vi "Post-Install Custom Action.vi"(10 "Variant":variant) -> (0 "error out":errorcluster)   [LabVIEW 2013]
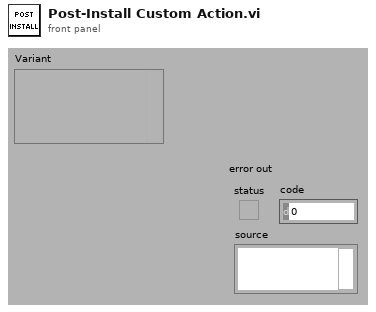
[diagram p1: front panel]
types:
  T1 = enum32{"invalid lock state", "Not Locked", "Locked (No Password)", "Password-protected"}
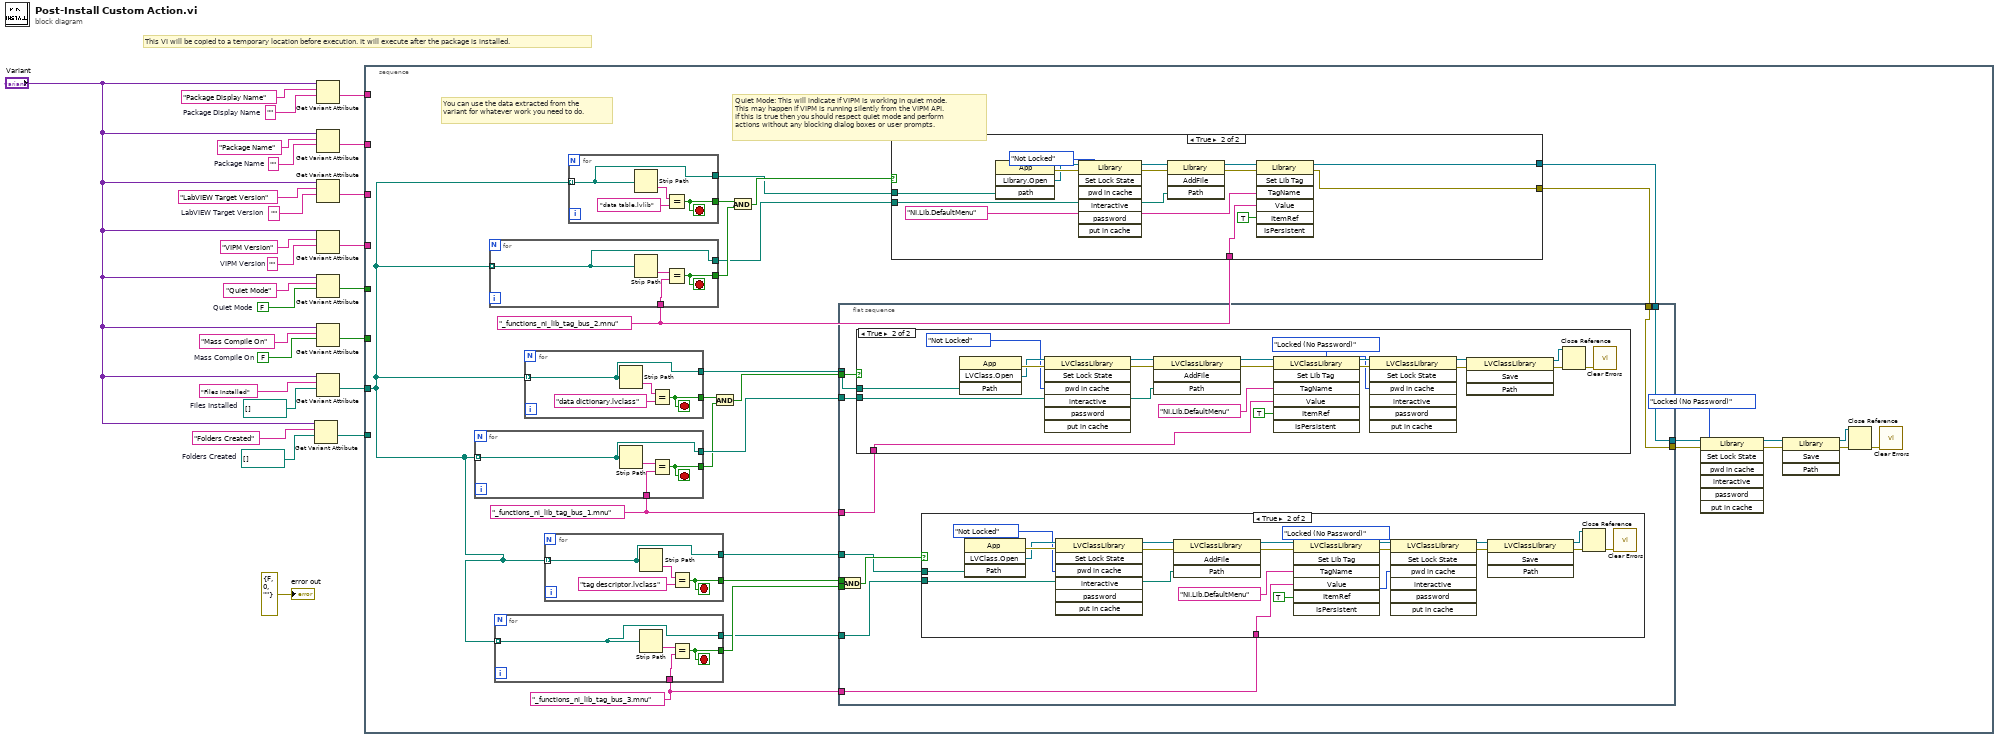
[diagram p0: block diagram]
diagram:
  w1 = path[] []  # Folders Created
  w2 = path[] []  # Files Installed
  w8 = FALSE  # Mass Compile On
  w9 = ""  # Package Display Name
  w16 = FALSE  # Quiet Mode
  w19 = ""  # VIPM Version
  w21 = ""  # LabVIEW Target Version
  w23 = ""  # Package Name
  # "This VI will be copied to a temporary location before execution. It will execute after the package is installed."
  n1 = Get Variant Attribute(Variant="Variant", name="Folders Created", default value (empty Variant)=w1) -> (value=w6:path[])  [unwired: 1 in, 3 out]
  n2 = Get Variant Attribute(Variant="Variant", name="Package Display Name", default value (empty Variant)=w9) -> (value=w15:string)  [unwired: 1 in, 3 out]
  n3 = Get Variant Attribute(Variant="Variant", name="Package Name", default value (empty Variant)=w23) -> (value=w14:string)  [unwired: 1 in, 3 out]
  n4 = Get Variant Attribute(Variant="Variant", name="LabVIEW Target Version", default value (empty Variant)=w21) -> (value=w13:string)  [unwired: 1 in, 3 out]
  n5 = Get Variant Attribute(Variant="Variant", name="VIPM Version", default value (empty Variant)=w19) -> (value=w12:string)  [unwired: 1 in, 3 out]
  n6 = Get Variant Attribute(Variant="Variant", name="Quiet Mode", default value (empty Variant)=w16) -> (value=w11:bool)  [unwired: 1 in, 3 out]
  n7 = Get Variant Attribute(Variant="Variant", name="Mass Compile On", default value (empty Variant)=w8) -> (value=w10:bool)  [unwired: 1 in, 3 out]
  n8 = Get Variant Attribute(Variant="Variant", name="Files Installed", default value (empty Variant)=w2) -> (value=w5:path[])  [unwired: 1 in, 3 out]
  n9 = stacked-sequence {
    tunnel: w15 -> [_]
    tunnel: w14 -> [_]
    tunnel: w13 -> [_]
    tunnel: w12 -> [_]
    tunnel: w11 -> [_]
    tunnel: w10 -> [_]
    tunnel: w5 -> [w40]
    tunnel: w6 -> [_]
    frame #0 {
      w37 = "_functions_ni_lib_tag_bus_3.mnu" ("pattern")
      w38 = "_functions_ni_lib_tag_bus_1.mnu" ("pattern")
      w39 = "_functions_ni_lib_tag_bus_2.mnu" ("pattern")
      # "Quiet Mode: This will indicate if VIPM is working in quiet mode.\nThis may happen if VIPM is running silently from the VIPM API.\nIf this is true then you should respect quiet mode and perform\nactions without any blocking dialog boxes or user prompts."
      # "You can use the data extracted from the variant for whatever work you need to do."
      n10 = for {
        tunnel: w40 -> [w115] mode=indexing
        tunnel: [w115] -> w49
        tunnel: [w117] -> w45
        tunnel: w38 -> [w116]
        stop <- w117 stop-if-true
        n11 = Strip Path(path=w115) -> (name=w118:string)  [unwired: 1 out]
        n12 = Equal?(x=w118, y=w116) -> (x = y?=w117:bool)
      }
      n13 = for {
        tunnel: w40 -> [w137] mode=indexing
        tunnel: [w137] -> w50
        tunnel: [w139] -> w54
        tunnel: w39 -> [w138]
        stop <- w139 stop-if-true
        n14 = Strip Path(path=w137) -> (name=w140:string)  [unwired: 1 out]
        n15 = Equal?(x=w140, y=w138) -> (x = y?=w139:bool)
      }
      n16 = for {
        tunnel: w40 -> [w107] mode=indexing
        tunnel: [w107] -> w41
        tunnel: [w109] -> w44
        tunnel: w37 -> [w108]
        stop <- w109 stop-if-true
        n17 = Strip Path(path=w107) -> (name=w110:string)  [unwired: 1 out]
        n18 = Equal?(x=w110, y=w108) -> (x = y?=w109:bool)
      }
      n19 = for {
        tunnel: w40 -> [w119] mode=indexing
        tunnel: [w119] -> w48
        tunnel: [w120] -> w46
        stop <- w120 stop-if-true
        n20 = Strip Path(path=w119) -> (name=w121:string)  [unwired: 1 out]
        n21 = Equal?(x=w121, y="data dictionary.lvclass" ("pattern")) -> (x = y?=w120:bool)
      }
      n22 = for {
        tunnel: w40 -> [w111] mode=indexing
        tunnel: [w111] -> w42
        tunnel: [w112] -> w43
        stop <- w112 stop-if-true
        n23 = Strip Path(path=w111) -> (name=w113:string)  [unwired: 1 out]
        n24 = Equal?(x=w113, y="tag descriptor.lvclass" ("pattern")) -> (x = y?=w112:bool)
      }
      n25 = for {
        tunnel: w40 -> [w141] mode=indexing
        tunnel: [w141] -> w51
        tunnel: [w142] -> w53
        stop <- w142 stop-if-true
        n26 = Strip Path(path=w141) -> (name=w143:string)  [unwired: 1 out]
        n27 = Equal?(x=w143, y="data table.lvlib" ("pattern")) -> (x = y?=w142:bool)
      }
      n28 = And(x=w46, y=w45) -> (x .and. y?=w47:bool)
      n29 = And(x=w53, y=w54) -> (x .and. y?=w52:bool)
      n30 = flat-sequence {
        tunnel: w49 -> [w66]
        tunnel: w48 -> [w65]
        tunnel: w47 -> [w64]
        tunnel: w44 -> [w63]
        tunnel: w43 -> [w62]
        tunnel: w42 -> [w60]
        tunnel: w41 -> [w59]
        tunnel: w38 -> [w58]
        tunnel: w37 -> [w57]
        tunnel: w31 -> [w55]
        tunnel: [w56] -> w30
        tunnel: w29 -> [w56]
        tunnel: [w55] -> w28
        frame #0 {
          n31 = And(x=w62, y=w63) -> (x .and. y?=w61:bool)
          n32 = case shown="True" w64 {
            tunnel: w65 -> [_ w97]
            tunnel: w66 -> [_ w96]
            tunnel: w58 -> [_ w95]
            frame False {
            }
            frame True {
              n33 = invoke class="App" method="LVClass.Open"("Path"=w97) -> (error out=w106:errorcluster, "LVClass.Open"=w90:refnum<vi>)  [unwired: 3 in, 2 out]
              n34 = invoke class="LVClassLibrary" method="Set Lock State"(reference=w90, error in=w106, "pwd in cache"=T1."Not Locked" ("lock state")) -> (reference out=w89:refnum<vi>, error out=w91:errorcluster)  [unwired: 4 in, 5 out]
              n35 = invoke class="LVClassLibrary" method="AddFile"(reference=w89, error in=w91, "Path"=w96) -> (reference out=w103:refnum<vi>, error out=w104:errorcluster)  [unwired: 1 in, 2 out]
              n36 = invoke class="LVClassLibrary" method="Set Lib Tag"(reference=w103, error in=w104, "TagName"="NI.Lib.DefaultMenu" ("Tag Name"), "Value"=w95, "ItemRef"=TRUE ("Is Persistent")) -> (reference out=w93:refnum<vi>, error out=w102:errorcluster)  [unwired: 2 in, 5 out]
              n37 = invoke class="LVClassLibrary" method="Set Lock State"(reference=w93, error in=w102, "pwd in cache"=T1."Locked (No Password)" ("lock state")) -> (reference out=w92:refnum<vi>, error out=w94:errorcluster)  [unwired: 4 in, 5 out]
              n38 = invoke class="LVClassLibrary" method="Save"(reference=w92, error in=w94) -> (reference out=w99:refnum<vi>, error out=w100:errorcluster)  [unwired: 2 in, 2 out]
              n39 = Close Reference(reference=w99, error in (no error)=w100) -> (error out=w105:errorcluster)
              n40 = call <vilib>:"Clear Errors.vi"("error in (no error)"=w105) -> ()  [unwired: 6 in, 1 out]
            }
          }
          n41 = case shown="True" w61 {
            tunnel: w60 -> [_ w77]
            tunnel: w59 -> [_ w76]
            tunnel: w57 -> [_ w75]
            frame False {
            }
            frame True {
              n42 = invoke class="App" method="LVClass.Open"("Path"=w77) -> (error out=w86:errorcluster, "LVClass.Open"=w70:refnum<vi>)  [unwired: 3 in, 2 out]
              n43 = invoke class="LVClassLibrary" method="Set Lock State"(reference=w70, error in=w86, "pwd in cache"=T1."Not Locked" ("lock state")) -> (reference out=w69:refnum<vi>, error out=w71:errorcluster)  [unwired: 4 in, 5 out]
              n44 = invoke class="LVClassLibrary" method="AddFile"(reference=w69, error in=w71, "Path"=w76) -> (reference out=w83:refnum<vi>, error out=w84:errorcluster)  [unwired: 1 in, 2 out]
              n45 = invoke class="LVClassLibrary" method="Set Lib Tag"(reference=w83, error in=w84, "TagName"="NI.Lib.DefaultMenu" ("Tag Name"), "Value"=w75, "ItemRef"=TRUE ("Is Persistent")) -> (reference out=w73:refnum<vi>, error out=w82:errorcluster)  [unwired: 2 in, 5 out]
              n46 = invoke class="LVClassLibrary" method="Set Lock State"(reference=w73, error in=w82, "pwd in cache"=T1."Locked (No Password)" ("lock state")) -> (reference out=w72:refnum<vi>, error out=w74:errorcluster)  [unwired: 4 in, 5 out]
              n47 = invoke class="LVClassLibrary" method="Save"(reference=w72, error in=w74) -> (reference out=w79:refnum<vi>, error out=w80:errorcluster)  [unwired: 2 in, 2 out]
              n48 = Close Reference(reference=w79, error in (no error)=w80) -> (error out=w85:errorcluster)
              n49 = call <vilib>:"Clear Errors.vi"("error in (no error)"=w85) -> ()  [unwired: 6 in, 1 out]
            }
          }
        }
      }
      n50 = case shown="True" w52 {
        tunnel: w51 -> [_ w131]
        tunnel: w50 -> [_ w130]
        tunnel: w39 -> [_ w129]
        tunnel: [_ w128] -> w31
        tunnel: [_ w127] -> w29
        frame False {
        }
        frame True {
          n51 = invoke class="App" method="Library.Open"("path"=w131) -> (error out=w136:errorcluster, "Open Library"=w125:refnum<vi>)  [unwired: 3 in, 2 out]
          n52 = invoke class="Library" method="Set Lock State"(reference=w125, error in=w136, "pwd in cache"=T1."Not Locked" ("lock state")) -> (reference out=w124:refnum<vi>, error out=w126:errorcluster)  [unwired: 4 in, 5 out]
          n53 = invoke class="Library" method="AddFile"(reference=w124, error in=w126, "Path"=w130) -> (reference out=w134:refnum<vi>, error out=w135:errorcluster)  [unwired: 1 in, 2 out]
          n54 = invoke class="Library" method="Set Lib Tag"(reference=w134, error in=w135, "TagName"="NI.Lib.DefaultMenu" ("Tag Name"), "Value"=w129, "ItemRef"=TRUE ("Is Persistent")) -> (reference out=w128:refnum<vi>, error out=w127:errorcluster)  [unwired: 2 in, 5 out]
        }
      }
      n55 = invoke class="Library" method="Set Lock State"(reference=w28, error in=w30, "pwd in cache"=T1."Locked (No Password)" ("lock state")) -> (reference out=w36:refnum<vi>, error out=w35:errorcluster)  [unwired: 4 in, 5 out]
      n56 = invoke class="Library" method="Save"(reference=w36, error in=w35) -> (reference out=w34:refnum<vi>, error out=w33:errorcluster)  [unwired: 2 in, 2 out]
      n57 = Close Reference(reference=w34, error in (no error)=w33) -> (error out=w32:errorcluster)
      n58 = call <vilib>:"Clear Errors.vi"("error in (no error)"=w32) -> ()  [unwired: 6 in, 1 out]
    }
  }
  "error out" <- errorcluster {"status"=FALSE, "code"=0, "source"=""} ("error out")
